vi "DependenciesUI.vi"() -> ()   [LabVIEW 2019, in "Dependencies.lvclass"]
uses:
  Dependencies.lvclass
  <vilib>/NI/Configuration Framework/Node/NodeRef.ctl
  <vilib>/NI/Configuration Framework/Node/NISE_CEF_Node.lvclass
  <vilib>/NI/AMC/Message Queue.ctl
  <vilib>/NI/AMC/Message.ctl
  <vilib>/NI/Tools/Keyed Array/KeyedArray.ctl
  <vilib>/NI/Configuration Framework/Node/UserEventRef.ctl
  <vilib>/NI/Configuration Framework/Controls/EventCluster.ctl
  XML Controls/Dependencies Properties.ctl
  XML Controls/Path Cluster.ctl
  XML Controls/Supported Targets.ctl
  C:/Program Files (x86)/National Instruments/LabVIEW 2019/vi.lib/NI/Configuration Framework/Node/NISE_CEF_Node.lvclass
  <vilib>/NI/AMC/Create Single Message.vi
  <vilib>/NI/AMC/Update Message Routing Info.vi
  <vilib>/NI/AMC/Send Message.vi
  <vilib>/NI/AMC/AMC.lvlib
  Configuration Tool.lvlib
  <vilib>/NI/Tools/Keyed Array/Tools_KeyedArray.lvlib
  <vilib>/NI/Configuration Framework/NISE_CEF_TreeControl.lvlib
  VeriStand Custom Device XML Parser.lvlib
panel:
  in  "Main UI Tab":enum32{"Dependencies"}(tab)
  in  "Multicolumn Listbox":i32(listbox)
  in  "Add New":bool
  out "All Dependencies Properties":T1[](array[typedef])
  in  "user event":T4
  in  "main queue":T5
  in  "node ref":T6
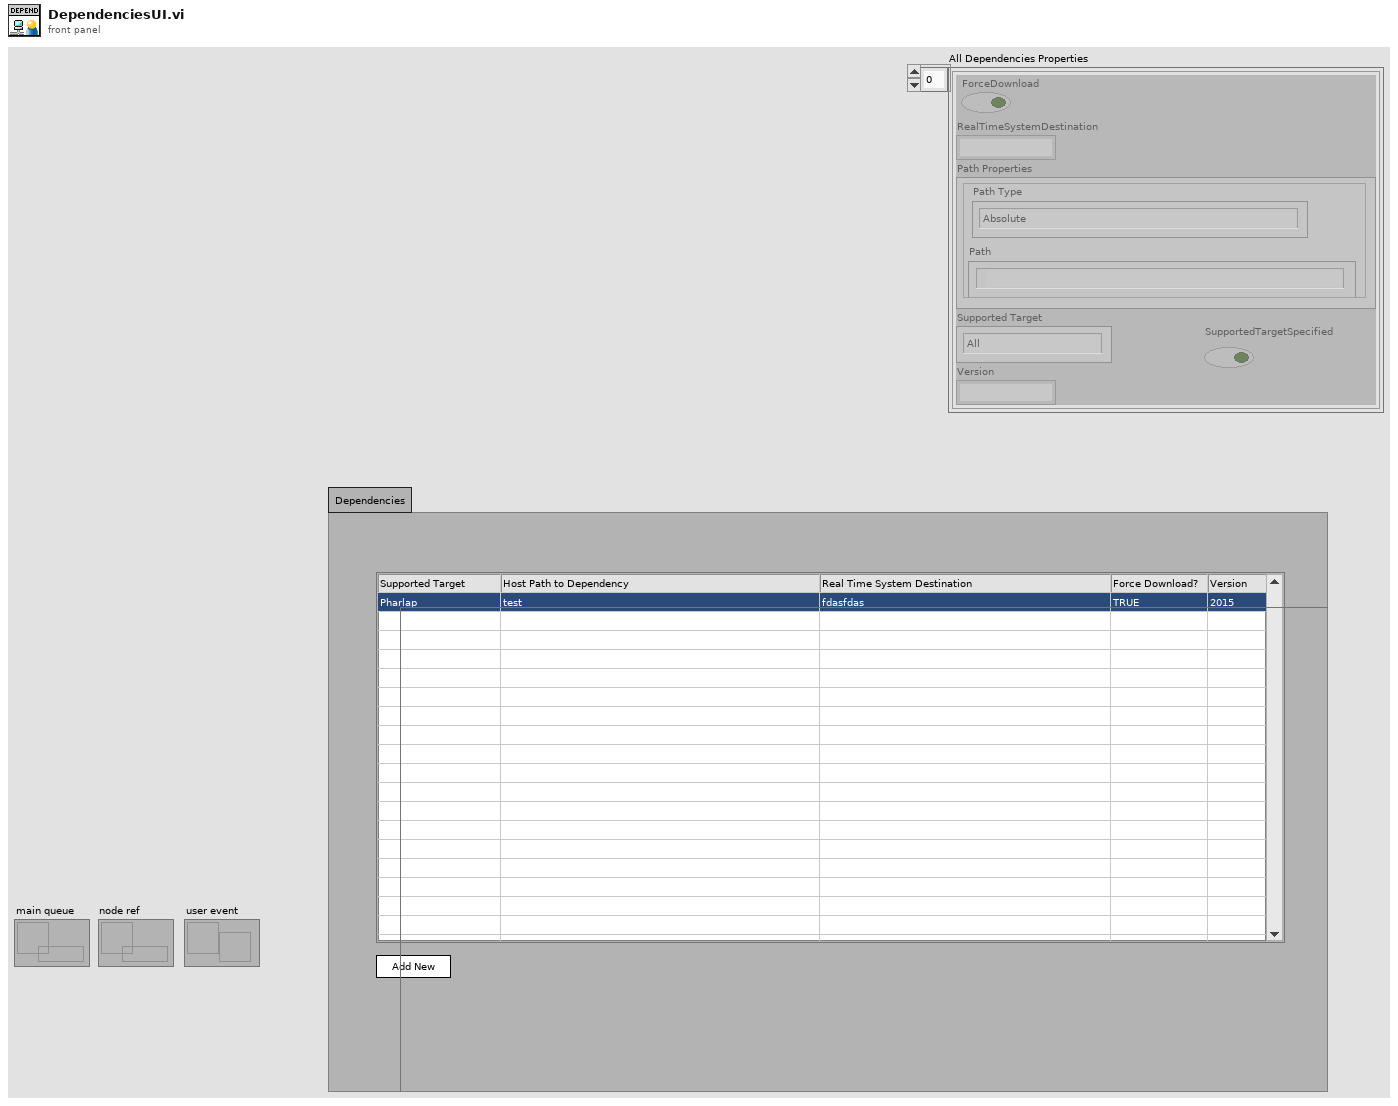
[diagram p1: front panel]
types:
  T1 = typedef "VeriStand Custom Device XML Parser.lvlib/Dependencies Properties.ctl" = cluster{"ForceDownload":bool, "RealTimeSystemDestination":string, "Path Properties":T2, "Supported Target":T3, "Version":string, "SupportedTargetSpecified":bool}
  T2 = typedef "VeriStand Custom Device XML Parser.lvlib/Path Cluster.ctl" = cluster{"Path":path, "Path Type":enum16{"Absolute", "To Base", "To Common Doc Dir", "To Application Data Dir"}}
  T3 = typedef "VeriStand Custom Device XML Parser.lvlib/Supported Targets.ctl" = enum16{"All", "Pharlap", "VxWorks", "Windows", "Linux_32_ARM", "Linux_x64", "PharlapWindows", "PharlapVxWorks", "VxWorksWindows"}
  T4 = typedef "NISE_CEF_Node.lvclass/UserEventRef.ctl" = refnum<user-event>
  T5 = typedef "AMC.lvlib/Message Queue.ctl" = refnum<queue>
  T6 = typedef "NISE_CEF_Node.lvclass/NodeRef.ctl" = refnum<data-value>
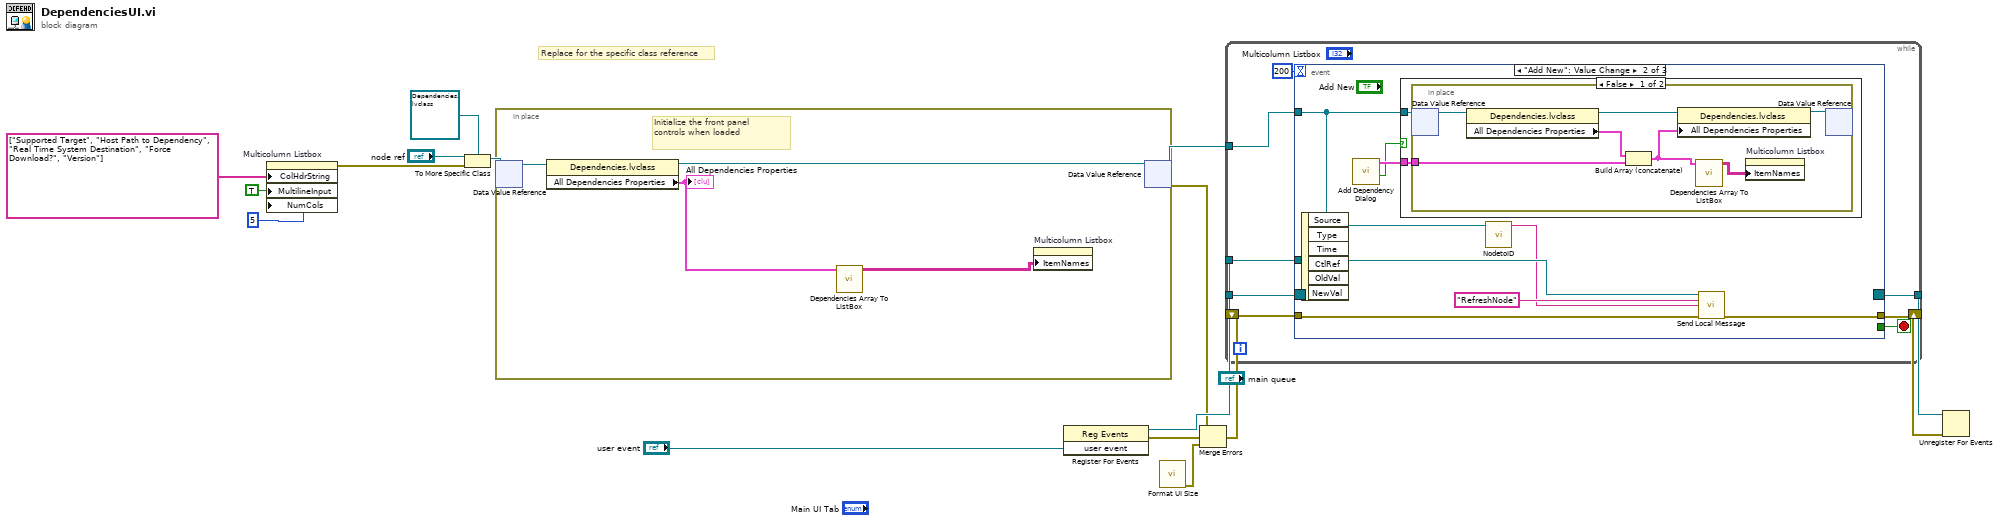
[diagram p0: block diagram]
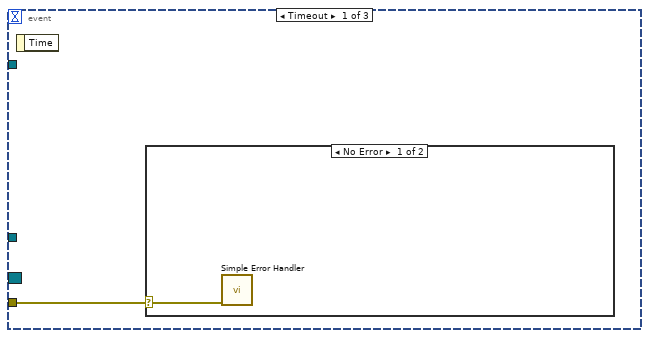
[diagram p2: hidden frame]
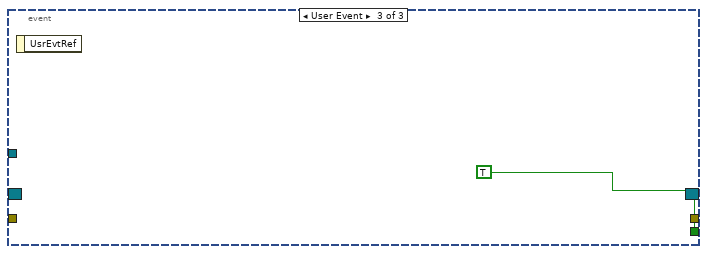
[diagram p5: hidden frame]
diagram:
  # "Replace for the specific class reference"
  n1 = property on="Multicolumn Listbox" class="MCListbox (strict)"("ColHdrString"=string[] ["Supported Target", "Host Path to Dependency", "Real Time System Destination", "Force Download?", "Version"] ("Column Header Strings[]"), "MultilineInput"=TRUE ("Multiple Line Input"), "NumCols"=u32 5 ("Number of Columns")) -> (error out=w2:errorcluster)  [unwired: 2 in, 1 out]
  n2 = To More Specific Class(target class=refnum<data-value> refnum ("data value reference"), reference="node ref", error in=w2) -> (specific class reference=w10:refnum<data-value>)  [unwired: 1 out]
  n3 = in-place {
    # "Initialize the front panel controls when loaded"
    n4 = in-place-dvr #1(w10) -> (w21:refnum<class "Dependencies.lvclass">)  [unwired: 1 out]
    n5 = property class="Dependencies.lvclass"(reference=w21) -> (reference out=w20:refnum<class "Dependencies.lvclass">, "All Dependencies Properties"=w19:T1[])  [unwired: 1 in, 1 out]
    "All Dependencies Properties" <- w19
    n6 = call "Dependencies Array To ListBox.vi"("All Dependencies Properties"=w19) -> ("Array"=w18:string[][])  [unwired: 10 in]
    n7 = property on="Multicolumn Listbox" class="MCListbox (strict)"("ItemNames"=w18) -> ()  [unwired: 2 in, 2 out]
    n8 = in-place-dvr #1(w20) -> (w17:refnum<data-value>, w7:errorcluster)
  }
  n9 = register-events("user event") -> (reference out=w14:refnum<event-registration>, error out=w8:errorcluster)  [unwired: 2 in]
  n10 = call "Format UI Size.vi"() -> ("error out"=w1:errorcluster)  [unwired: 11 in]
  n11 = Merge Errors(w7, w8, w1) -> (w6:errorcluster)
  n12 = while {
    tunnel: w17 -> [w29]
    tunnel: "main queue" -> [w28]
    tunnel: w14 -> [w26]
    tunnel: [w25] -> w13
    shift-right: [w23] -> w12
    shift-left: w6 -> [w22]
    stop <- w24 stop-if-true
    n13 = event shown="[1] \"Add New\": Value Change" {
      selector: w26 -> [_ _ _]
      dyn-events: [_ _ _] -> w25
      timeout: 200 -> [_ _ _]
      tunnel: w29 -> [_ w37 _]
      tunnel: w28 -> [_ w38 _]
      tunnel: [_ _ TRUE] -> w24
      tunnel: [_ w35 _] -> w23
      tunnel: w22 -> [w30 w34 _]
      event Timeout {
        n14 = event-data() -> ()  [unwired: 1 in, 1 out]
        n15 = case shown="No Error" w30 {
          selector: w30 -> [w31 _]
          frame No Error {
            n16 = call <vilib>:"Simple Error Handler.vi"("error in (no error)"=w31) -> ()  [unwired: 4 in, 5 out]
          }
          frame Error {
          }
        }
      }
      event "Add New": Value Change {
        n17 = event-data() -> ()  [unwired: 1 in, 6 out]
        n18 = call "Add Dependency Dialog.vi"() -> ("Cancelled?"=w32:bool, "Dependency Out"=w33:T1)  [unwired: 10 in]
        n19 = case shown="False" w32 {
          tunnel: w37 -> [w41 _]
          tunnel: w33 -> [w40 _]
          frame False {
            n20 = in-place {
              in-place-border: w40 -> [w44]
              n21 = in-place-dvr #2(w41) -> (w47:refnum<class "Dependencies.lvclass">)  [unwired: 1 out]
              n22 = property class="Dependencies.lvclass"(reference=w47) -> (reference out=w46:refnum<class "Dependencies.lvclass">, "All Dependencies Properties"=w45:T1[])  [unwired: 1 in, 1 out]
              n23 = Build Array (concatenate)(w45, w44) -> (w43:T1[])
              n24 = property class="Dependencies.lvclass"(reference=w46, "All Dependencies Properties"=w43) -> (reference out=w48:refnum<class "Dependencies.lvclass">)  [unwired: 1 in, 1 out]
              n25 = call "Dependencies Array To ListBox.vi"("All Dependencies Properties"=w43) -> ("Array"=w42:string[][])  [unwired: 10 in]
              n26 = property on="Multicolumn Listbox" class="MCListbox (strict)"("ItemNames"=w42) -> ()  [unwired: 2 in, 2 out]
              n27 = in-place-dvr #2(w48) -> ()  [unwired: 2 out]
            }
          }
          frame True {
          }
        }
        n28 = call <vilib>:"NodetoID.vi"("node ref"=w37) -> ("ID"=w36:string)  [unwired: 9 in, 1 out]
        n29 = call <vilib>:"Send Local Message.vi"("message queue in"=w38, "message name"="RefreshNode" ("Message Name"), "message value"=w36, "error in"=w34) -> ("error out"=w35:errorcluster)  [unwired: 9 in, 2 out]
      }
      event User Event {
        n30 = event-data() -> ()  [unwired: 1 in, 1 out]
      }
    }
  }
  n31 = Unregister For Events(event registration refnum=w13, error in=w12) -> ()  [unwired: 1 out]
